vi "Add Block Diagram Content.vi"(8 "error in (no error)":errorcluster, 10 "ModuleLoop":T1, 11 "FPGA Addon Output in":refnum<class "FPGA Addon Output.lvclass">) -> (0 "error out":errorcluster, 2 "Term Refnum":refnum<vi>, 3 "FPGA Addon Output out":refnum<class "FPGA Addon Output.lvclass">)   [LabVIEW 2015, in "FPGA Addon Output.lvclass"]
uses:
  FPGA Addon Output.lvclass
  VI/VI/Module.Refs.ctl
  <vilib>/Utility/miscctls.llb/LVPointTypeDef.ctl
  Signal/Read IP Core Path.vi
  Signal/Read Signal Name.vi
  VI/Structures/Structures.lvclass
  VI/VI/VI.lvclass
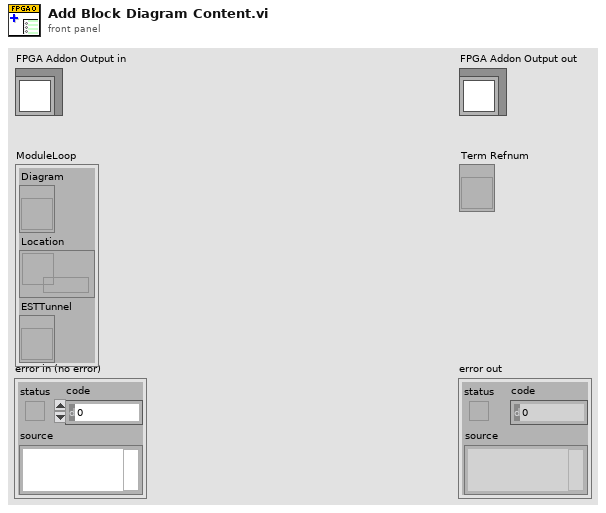
[diagram p1: front panel]
types:
  T1 = typedef "VI.lvclass/Module.Refs.ctl" = cluster{"Diagram":refnum<vi>, "Location":refnum<data-value>, "ESTTunnel":refnum<vi>}
  T2 = typedef "LVPointTypeDef.ctl" = cluster{"Horizontal":i16, "Vertical":i16}
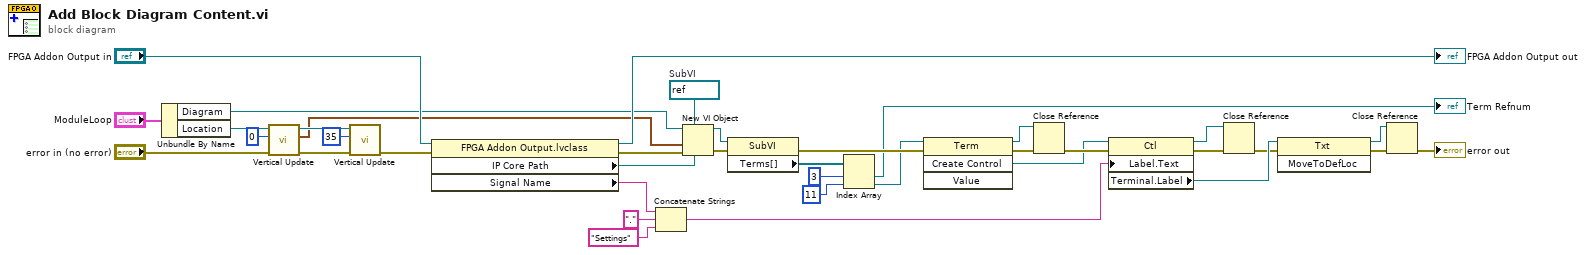
[diagram p0: block diagram]
diagram:
  w16 = refnum<vi> refnum  # SubVI
  n1 = Unbundle By Name("ModuleLoop") -> ("Diagram"=w1:refnum<vi>, "Location"=w34:refnum<data-value>)
  n2 = call "Vertical Update.vi"("error in (no error)"="error in (no error)", "Vertical Change"=i16 0, "Location"=w34) -> ("error out"=w30:errorcluster, "location out"=w2:T2, "Location"=w32:refnum<data-value>)  [unwired: 6 in]
  n3 = call "Vertical Update.vi"("error in (no error)"=w30, "Vertical Change"=i16 35, "Location"=w32) -> ("error out"=w29:errorcluster)  [unwired: 6 in, 2 out]
  n4 = property class="FPGA Addon Output.lvclass"(reference="FPGA Addon Output in", error in=w29) -> (reference out=→"FPGA Addon Output out":refnum<class "FPGA Addon Output.lvclass">, error out=w7:errorcluster, "IP Core Path"=w3:path, "Signal Name"=w4:string)
  n5 = Concatenate Strings(w4, "." ("string"), "Settings" ("string")) -> (w23:string)
  n6 = New VI Object(vi object class=w16, owner refnum=w1, position/next to=w2, 6:w3, 8:w7) -> (object refnum=w20:refnum<vi>, 0:w21:errorcluster)  [unwired: 3 in]
  n7 = property class="SubVI"(reference=w20, error in=w21) -> (error out=w22:errorcluster, "Terms[]"=w17:refnum<vi>[])  [unwired: 1 out]
  n8 = Index Array(array=w17, index #1=3 ("index"), index #2=11 ("index")) -> (element #1=→"Term Refnum":refnum<vi>, element #2=w8:refnum<vi>)
  n9 = invoke class="Term" method="Create Control"(reference=w8, error in=w22) -> (reference out=w27:refnum<vi>, error out=w26:errorcluster, "Create Control"=w15:refnum<vi>)  [unwired: 2 in, 1 out]
  n10 = Close Reference(reference=w27, error in (no error)=w26) -> (error out=w28:errorcluster)
  n11 = property class="Ctl"(reference=w15, error in=w28, "Label.Text"=w23) -> (reference out=w14:refnum<vi>, error out=w12:errorcluster, "Terminal.Label"=w13:refnum<vi>)
  n12 = Close Reference(reference=w14, error in (no error)=w12) -> (error out=w11:errorcluster)
  n13 = invoke class="Txt" method="MoveToDefLoc"(reference=w13, error in=w11) -> (reference out=w9:refnum<vi>, error out=w10:errorcluster)  [unwired: 1 in, 1 out]
  n14 = Close Reference(reference=w9, error in (no error)=w10) -> (error out=→"error out":errorcluster)
